vi "LED Tester.vi"   [LabVIEW 2014]
uses:
  LED Values.vi
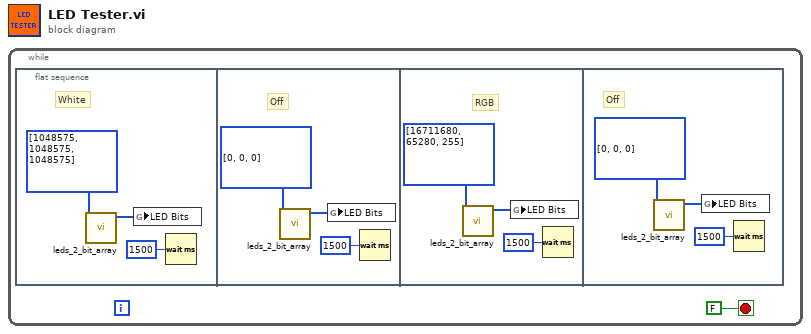
[diagram p0: block diagram]
diagram:
  n1 = while {
    stop <- FALSE stop-if-true
    n2 = flat-sequence {
      frame #0 {
        # "White"
        n3 = call "leds_2_bit_array.vi"("LEDs"=i32[] [1048575, 1048575, 1048575]) -> ("Bit Array"=w3:u8[])  [unwired: 10 in]
        n4 = global write "LED Values.vi" "LED Bits"(w3) -> ()
        n5 = Wait (ms)(milliseconds to wait=u32 1500) -> ()  [unwired: 1 out]
      }
      frame #1 {
        # "Off"
        n6 = call "leds_2_bit_array.vi"("LEDs"=i32[] [0, 0, 0]) -> ("Bit Array"=w6:u8[])  [unwired: 10 in]
        n7 = global write "LED Values.vi" "LED Bits"(w6) -> ()
        n8 = Wait (ms)(milliseconds to wait=u32 1500) -> ()  [unwired: 1 out]
      }
      frame #2 {
        # "RGB"
        n9 = call "leds_2_bit_array.vi"("LEDs"=i32[] [16711680, 65280, 255]) -> ("Bit Array"=w9:u8[])  [unwired: 10 in]
        n10 = global write "LED Values.vi" "LED Bits"(w9) -> ()
        n11 = Wait (ms)(milliseconds to wait=u32 1500) -> ()  [unwired: 1 out]
      }
      frame #3 {
        # "Off"
        n12 = call "leds_2_bit_array.vi"("LEDs"=i32[] [0, 0, 0]) -> ("Bit Array"=w12:u8[])  [unwired: 10 in]
        n13 = global write "LED Values.vi" "LED Bits"(w12) -> ()
        n14 = Wait (ms)(milliseconds to wait=u32 1500) -> ()  [unwired: 1 out]
      }
    }
  }
